vi "Set Ramp.vi"(8 "error in (no error)":errorcluster, 9 "Output #":i32=1, 10 "Ramp rate (0: off)":dbl, 11 "LakeShore T Controller Driver in":refnum<class "LakeShore T Controller Driver.lvclass">) -> (0 "error out":errorcluster, 3 "LakeShore T Controller Driver out":refnum<class "LakeShore T Controller Driver.lvclass">)   [LabVIEW 2021, in "LakeShore T Controller Driver.lvclass"]
uses:
  LakeShore T Controller Driver.lvclass
  LakeShore T Controller Driver.lvclass/LakeShore T Controller Driver.ctl
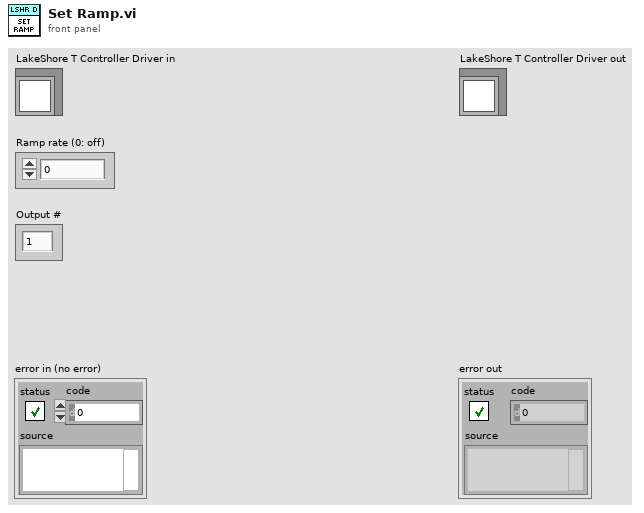
[diagram p1: front panel]
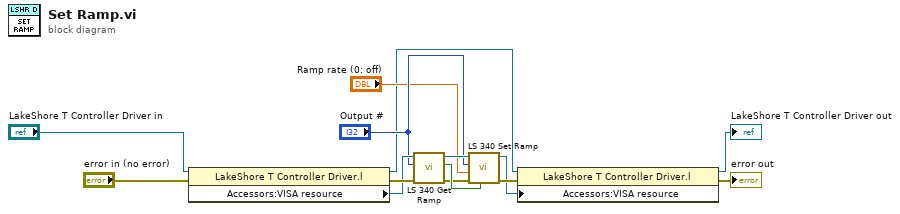
[diagram p0: block diagram]
diagram:
  n1 = property class="LakeShore T Controller Driver.l"(reference="LakeShore T Controller Driver in", error in="error in (no error)") -> (reference out=w6:refnum<class "LakeShore T Controller Driver.lvclass">, error out=w14:errorcluster, "Accessors:VISA resource"=w13:refnum<visa-resource-name>)
  n2 = call "LS 340 Get Ramp.vi"("error in (no error)"=w14, "Output #"="Output #", "VISA resource name"=w13) -> ("error out"=w8:errorcluster, "Ramp on"=w9:bool, "VISA Resource Name Out"=w12:refnum<visa-resource-name>)  [unwired: 5 in, 1 out]
  n3 = call "LS 340 Set Ramp.vi"("Ramp on"=w9, "error in (no error)"=w8, "Ramp rate, K/min"="Ramp rate (0: off)", "Output #"="Output #", "VISA resource name"=w12) -> ("error out"=w7:errorcluster, "VISA Resource Name Out"=w1:refnum<visa-resource-name>)  [unwired: 5 in]
  n4 = property class="LakeShore T Controller Driver.l"(reference=w6, error in=w7, "Accessors:VISA resource"=w1) -> (reference out=→"LakeShore T Controller Driver out":refnum<class "LakeShore T Controller Driver.lvclass">, error out=→"error out":errorcluster)
